vi "Create.vi"(8 "error in (no error)":errorcluster, 10 "Starting Values (Empty)":map{T1, T2}(c390)) -> (0 "error out":errorcluster, 3 "Tree Map out":refnum<class "Project Tree Map.lvclass">)   [LabVIEW 2020, in "VI Properties Editor.lvlib" / "Project Tree Map.lvclass"]
doc: "Creates the tree map."
uses:
  Project Tree Map.lvclass
  Tree Key.ctl
  Tree Entry.ctl
  Project Tree Map.lvclass/Project Tree Map.ctl
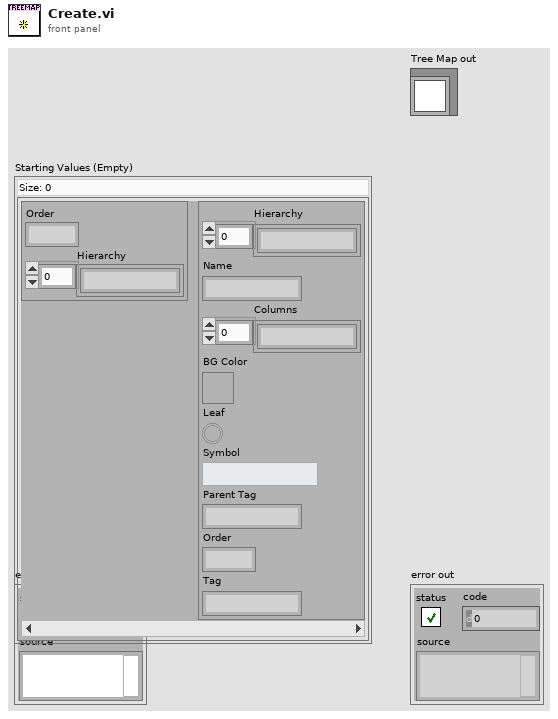
[diagram p1: front panel]
types:
  T1 = typedef "VI Properties Editor.lvlib/Project Tree Map.lvclass/Tree Key.ctl" = cluster{"Order":i32, "Hierarchy":string[]}
  T2 = typedef "VI Properties Editor.lvlib/Project Tree Map.lvclass/Tree Entry.ctl" = cluster{"Hierarchy":string[], "Name":string, "Columns":string[], "BG Color":u32, "Leaf":bool, "Symbol":string, "Parent Tag":string, "Order":i32, "Tag":string}
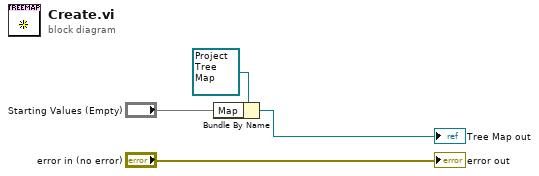
[diagram p0: block diagram]
diagram:
  n1 = Bundle By Name(cluster=refnum<class "Project Tree Map.lvclass"> refnum ("Tree Map in"), "Map"="Starting Values (Empty)") -> (→"Tree Map out":refnum<class "Project Tree Map.lvclass">)
  "error out" <- "error in (no error)"
